vi "DUT Info.vi"(10 "PORT CONFIGURATION":T3(array[cluster]), 11 "DUT Info":T1={"DUT IP"="192.168.1.12", "DUT Username"="Administrator", "DUT Password"="NITEST", "DUT SSH PORT"=22, "DUT iPERF TEST PORT"=0, "DUT MAC ADDRESS"="02:00:08:38:2d:37"}) -> (2 "destination MAC address":cluster{u8, u8, u8, u8, u8, u8}, 3 "Ping Addresses":T2[](array[typedef]))   [LabVIEW 2026]
uses:
  emea-tra-SSH_onRT_over_XNET_IPstack/DiagnosticModule/Ping/Controls/ECUAddress.ctl
  emea-tra-SSH_onRT_over_XNET_IPstack/DiagnosticModule/DiagnosticModule.lvlib
  DUT Info.ctl
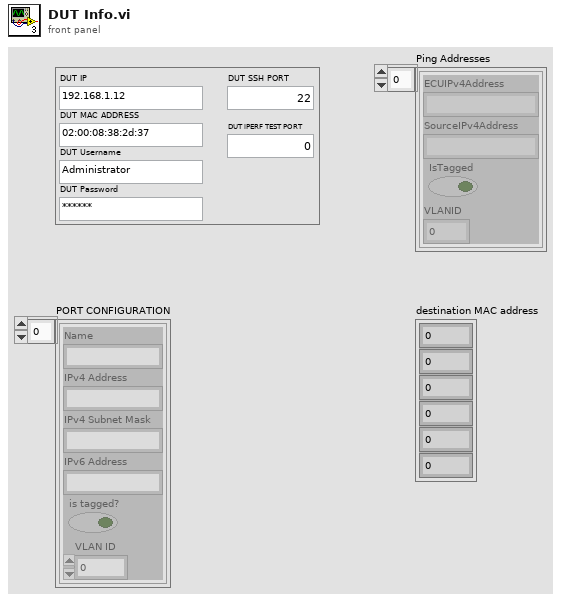
[diagram p1: front panel]
types:
  T1 = typedef "DUT Info.ctl" = cluster{"DUT IP":string, "DUT Username":string, "DUT Password":string, "DUT SSH PORT":u16, "DUT iPERF TEST PORT":u16, "DUT MAC ADDRESS":string}
  T2 = typedef "DiagnosticModule.lvlib/ECUAddress.ctl" = cluster{"ECUIPv4Address":string, "SourceIPv4Address":string, "IsTagged":bool, "VLANID":u16}
  T3 = cluster{"Name":string, "IPv4 Address":string, "IPv4 Subnet Mask":string, "IPv6 Address":string, "is tagged?":bool, "VLAN ID":u16}[]
  T4 = cluster{"Name":string, "IPv4 Address":string, "IPv4 Subnet Mask":string, "IPv6 Address":string, "is tagged?":bool, "VLAN ID":u16}
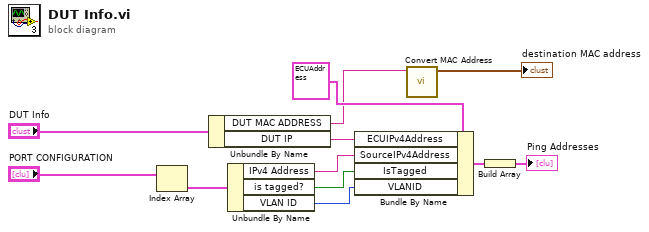
[diagram p0: block diagram]
diagram:
  n1 = Index Array(array="PORT CONFIGURATION") -> (element=w8:T4)  [unwired: 1 in]
  n2 = Unbundle By Name("DUT Info") -> ("DUT MAC ADDRESS"=w1:string, "DUT IP"=w2:string)
  n3 = Unbundle By Name(w8) -> ("IPv4 Address"=w9:string, "is tagged?"=w10:bool, "VLAN ID"=w11:u16)
  n4 = Bundle By Name(cluster=T2 {"ECUIPv4Address"="192.168.11.100", "SourceIPv4Address"="192.168.11.90", "IsTagged"=FALSE, "VLANID"=0} ("ECUAddress"), "ECUIPv4Address"=w2, "SourceIPv4Address"=w9, "IsTagged"=w10, "VLANID"=w11) -> (w5:T2)
  n5 = call "Convert MAC Address.vi"("DUT MAC ADDRESS"=w1) -> ("destination MAC address"=→"destination MAC address":cluster{u8, u8, u8, u8, u8, u8})  [unwired: 10 in]
  n6 = Build Array(w5) -> (→"Ping Addresses":T2[])
